vi "SwerveOdometry_UpdateWithTime4.vi"(4 "gyroAngle":T2={"VALUE"=0.0, "COS"=1.0, "SIN"=0.0} {"SIN" format="%13.4f"; "COS" format="%13.4f"; "VALUE" format="%13.4f"}, 5 "SWERVE_DRIVE_KINEMATICS":T3 {"PrevCoR"."Y" format="%14.3f"; "PrevCoR"."X" format="%14.3f"; "Modules"."Y" format="%14.3f"; "Modules"."X" format="%14.3f"}, 6 "Time":dbl, 7 "in SWERVE_DRIVE_ODOMETRY":T7={"POSE"={"TRANSLATION"={"X"=0.0, "Y"=0.0}, "ROTATION"={"VALUE"=0.0, "COS"=1.0, "SIN"=0.0}}, "GyroOffset"={"VALUE"=0.0, "COS"=1.0, "SIN"=0.0}, "PreviousAngle"={"VALUE"=0.0, "COS"=1.0, "SIN"=0.0}, "PrevTime"=0.0} {"PreviousAngle"."SIN" format="%13.4f"; "PreviousAngle"."COS" format="%13.4f"; "PreviousAngle"."VALUE" format="%13.4f"; "GyroOffset"."SIN" format="%13.4f"; "GyroOffset"."COS" format="%13.4f"; "GyroOffset"."VALUE" format="%13.4f"; "POSE"."ROTATION"."SIN" format="%13.4f"; "POSE"."ROTATION"."COS" format="%13.4f"; "POSE"."ROTATION"."VALUE" format="%13.4f"; "POSE"."TRANSLATION"."Y" format="%14.3f"; "POSE"."TRANSLATION"."X" format="%14.3f"}, 8 "Wheel State 3":T1={"Speed"=0.0, "Angle"={"VALUE"=0.0, "COS"=1.0, "SIN"=0.0}} {"Angle"."SIN" format="%13.4f"; "Angle"."COS" format="%13.4f"; "Angle"."VALUE" format="%13.4f"}, 9 "Wheel State 2":T1={"Speed"=0.0, "Angle"={"VALUE"=0.0, "COS"=1.0, "SIN"=0.0}} {"Angle"."SIN" format="%13.4f"; "Angle"."COS" format="%13.4f"; "Angle"."VALUE" format="%13.4f"}, 10 "Wheel State 1":T1={"Speed"=0.0, "Angle"={"VALUE"=0.0, "COS"=1.0, "SIN"=0.0}} {"Angle"."SIN" format="%13.4f"; "Angle"."COS" format="%13.4f"; "Angle"."VALUE" format="%13.4f"}, 11 "Wheel State 0":T1={"Speed"=0.0, "Angle"={"VALUE"=0.0, "COS"=1.0, "SIN"=0.0}} {"Angle"."SIN" format="%13.4f"; "Angle"."COS" format="%13.4f"; "Angle"."VALUE" format="%13.4f"}) -> (1 "robot POSE":T6={"TRANSLATION"={"X"=0.0, "Y"=0.0}, "ROTATION"={"VALUE"=0.0, "COS"=1.0, "SIN"=0.0}} {"ROTATION"."SIN" format="%13.4f"; "ROTATION"."COS" format="%13.4f"; "ROTATION"."VALUE" format="%13.4f"; "TRANSLATION"."Y" format="%14.3f"; "TRANSLATION"."X" format="%14.3f"}, 3 "out SWERVE_DRIVE_ODOMETRY":T7={"POSE"={"TRANSLATION"={"X"=0.0, "Y"=0.0}, "ROTATION"={"VALUE"=0.0, "COS"=1.0, "SIN"=0.0}}, "GyroOffset"={"VALUE"=0.0, "COS"=1.0, "SIN"=0.0}, "PreviousAngle"={"VALUE"=0.0, "COS"=1.0, "SIN"=0.0}, "PrevTime"=0.0} {"PreviousAngle"."SIN" format="%13.4f"; "PreviousAngle"."COS" format="%13.4f"; "PreviousAngle"."VALUE" format="%13.4f"; "GyroOffset"."SIN" format="%13.4f"; "GyroOffset"."COS" format="%13.4f"; "GyroOffset"."VALUE" format="%13.4f"; "POSE"."ROTATION"."SIN" format="%13.4f"; "POSE"."ROTATION"."COS" format="%13.4f"; "POSE"."ROTATION"."VALUE" format="%13.4f"; "POSE"."TRANSLATION"."Y" format="%14.3f"; "POSE"."TRANSLATION"."X" format="%14.3f"})   [LabVIEW 2019, in "Trajectory_Library.lvlib"]
doc: "Updates the robot's position on the field using forward kinematics and integration of the pose over time. This method takes in the current time as a parameter to calculate period (difference between two timestamps). The period is used to calculate the change in distance from a velocity. Thisalso takes in an angle parameter which is used instead of the angular rate that is calculated from forward kinematics.\n\nThis subVI is customized for 4 swerve modules.\n\nParameters:\n - InSwerveDriveOdometry - This data structure \n - currentTime - The current time in seconds.\n - gyroAngle - The angle reported by the gyroscope.\n - moduleState 0 - The current state of a swerve module. Please provide the states in the same order in which you instantiated your SwerveDriveKinematics.\n - moduleState 1 - The current state of a swerve module. \n - moduleState 2 - The current state of a swerve module. \n - moduleState 3 - The current state of a swerve module. \n\nReturns:\n - OutSwerveDriveOdometry - Updated data structure\n - The new pose of the robot."
uses:
  Trajectory_Library.lvlib
  TypeDef/ROTATION2D.ctl
  TypeDef/SWERVE_DRIVE_ODOMETRY.ctl
  TypeDef/POSE2D.ctl
  TypeDef/TRANSLATION2D.ctl
  TypeDef/SWERVE_DRIVE_KINEMATICS.ctl
  <vilib>/Analysis/Matrix/Datatypes/RealMatrix.ctl
  TypeDef/SWERVE_DRIVE_MODULE_STATE.ctl
  <vilib>/Analysis/Matrix/NI_Matrix.lvlib
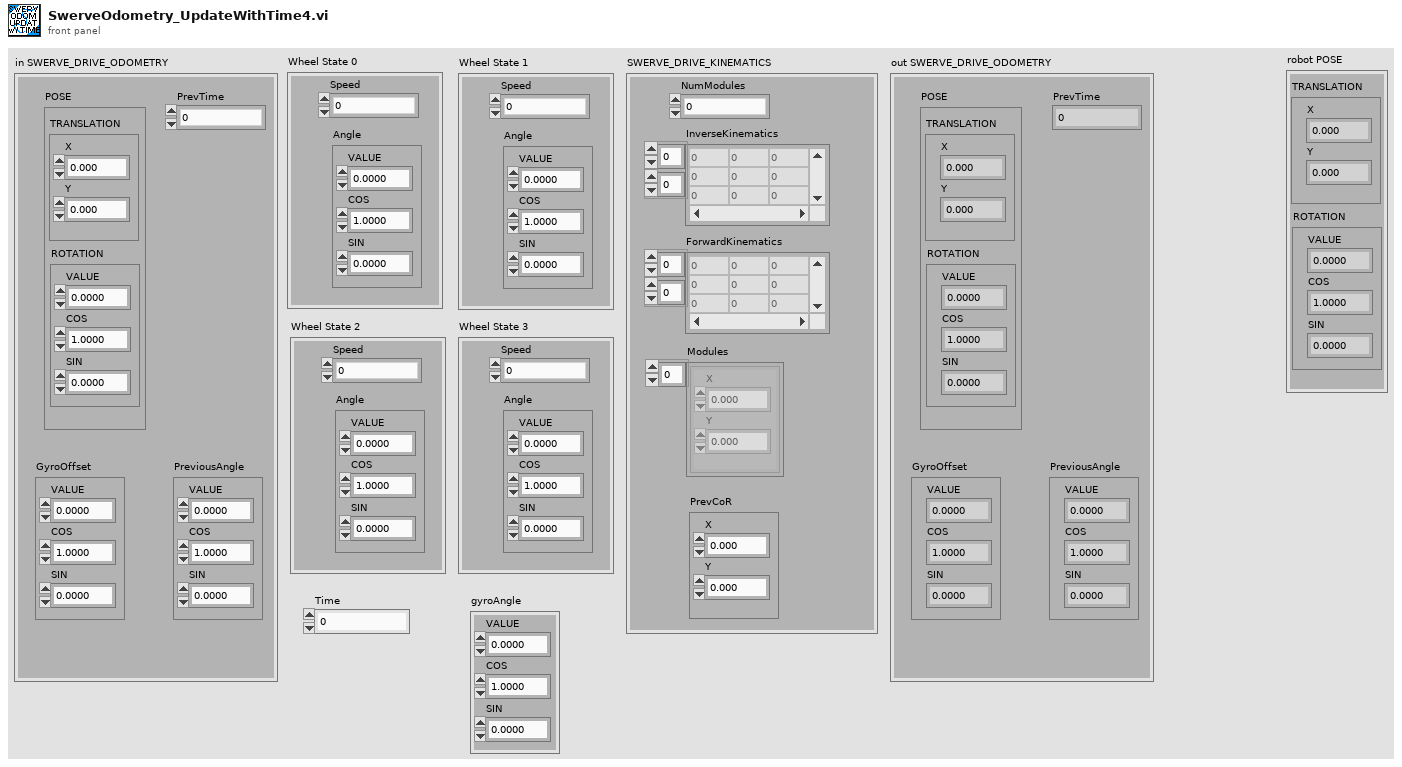
[diagram p1: front panel]
types:
  T1 = typedef "Trajectory_Library.lvlib/SWERVE_DRIVE_MODULE_STATE.ctl" = cluster{"Speed":dbl, "Angle":T2}
  T2 = typedef "Trajectory_Library.lvlib/ROTATION2D.ctl" = cluster{"VALUE":dbl, "COS":dbl, "SIN":dbl}
  T3 = typedef "Trajectory_Library.lvlib/SWERVE_DRIVE_KINEMATICS.ctl" = cluster{"NumModules":i32, "InverseKinematics":T4, "ForwardKinematics":T4, "Modules":T5[], "PrevCoR":T5}
  T4 = typedef "NI_Matrix.lvlib/RealMatrix.ctl" = dbl[][]
  T5 = typedef "Trajectory_Library.lvlib/TRANSLATION2D.ctl" = cluster{"X":dbl, "Y":dbl}
  T6 = typedef "Trajectory_Library.lvlib/POSE2D.ctl" = cluster{"TRANSLATION":T5, "ROTATION":T2}
  T7 = typedef "Trajectory_Library.lvlib/SWERVE_DRIVE_ODOMETRY.ctl" = cluster{"POSE":T6, "GyroOffset":T2, "PreviousAngle":T2, "PrevTime":dbl}
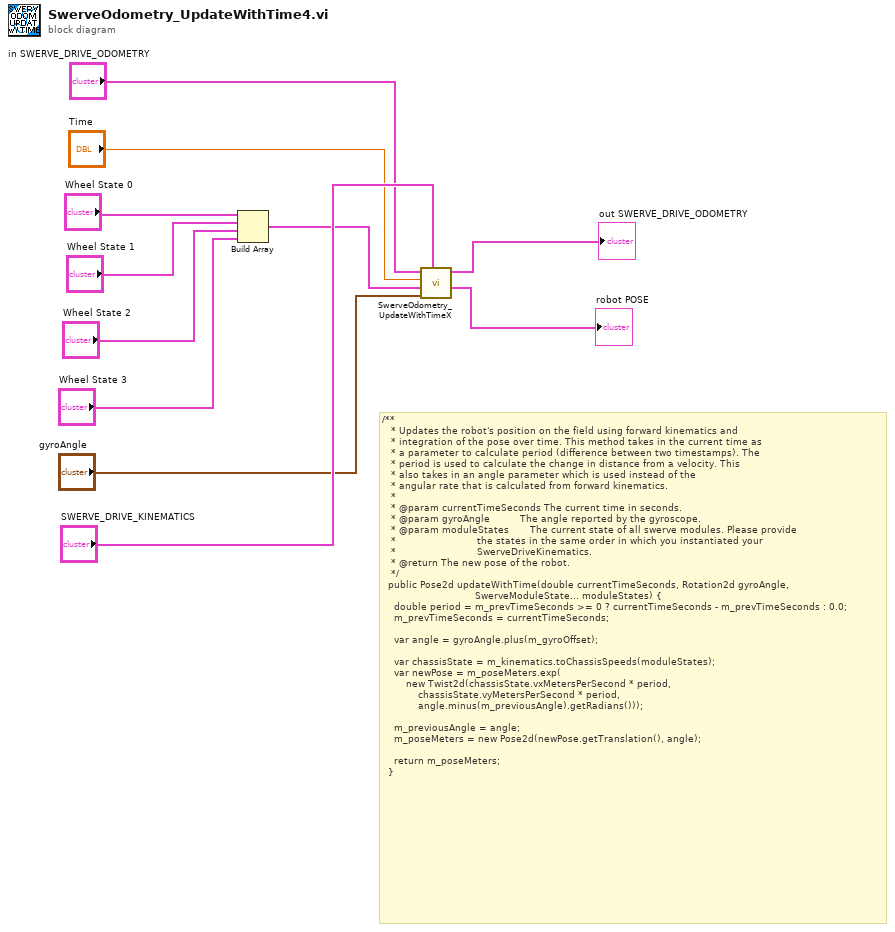
[diagram p0: block diagram]
diagram:
  # "/**\n   * Updates the robot's position on the field using forward kinematics and\n   * integration of the pose over time. This method takes in the current time as\n   * a parameter to calculate period (difference between two timestamps). The\n   * period is used to calculate the change in distance from a velocity. This\n   * also takes in an angle parameter which is used instead of the\n   * angular rate that is calculated from forward kinematics.\n   *\n   * @param currentTimeSeconds The current time in seconds.\n   * @param gyroAngle          The angle reported by the gyroscope.\n   * @param moduleStates       The current state of all swerve modules. Please provide\n   *                           the states in the same order in which you instantiated your\n   *                           SwerveDriveKinematics.\n   * @return The new pose of the robot.\n   */\n  public Pose2d updateWithTime(double currentTimeSeconds, Rotation2d gyroAngle,\n                               SwerveModuleState... moduleStates) {\n    double period = m_prevTimeSeconds >= 0 ? currentTimeSeconds - m_prevTimeSeconds : 0.0;\n    m_prevTimeSeconds = currentTimeSeconds;\n\n    var angle = gyroAngle.plus(m_gyroOffset);\n\n    var chassisState = m_kinematics.toChassisSpeeds(moduleStates);\n    var newPose = m_poseMeters.exp(\n        new Twist2d(chassisState.vxMetersPerSecond * period,\n            chassisState.vyMetersPerSecond * period,\n            angle.minus(m_previousAngle).getRadians()));\n\n    m_previousAngle = angle;\n    m_poseMeters = new Pose2d(newPose.getTranslation(), angle);\n\n    return m_poseMeters;\n  }"
  n1 = Build Array("Wheel State 0", "Wheel State 1", "Wheel State 2", "Wheel State 3") -> (w1:T1[])
  n2 = call "SwerveOdometry_UpdateWithTimeX.vi"("SWERVE_DRIVE_KINEMATICS"="SWERVE_DRIVE_KINEMATICS", "gyroAngle"="gyroAngle", "module States"=w1, "Time"="Time", "in SWERVE_DRIVE_ODOMETRY"="in SWERVE_DRIVE_ODOMETRY") -> ("robot POSE"=→"robot POSE":T6, "out SWERVE_DRIVE_ODOMETRY"=→"out SWERVE_DRIVE_ODOMETRY":T7)  [unwired: 5 in]
